vi "RawAttrMap.vi"() -> (3 "AttrMap":T1)   [LabVIEW 2019]
uses:
  Typedef/Def-AttrMap.ctl
  Typedef/Def-NameMap.ctl
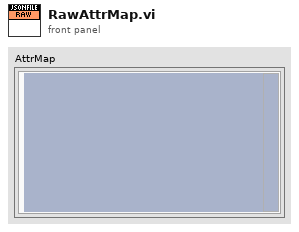
[diagram p1: front panel]
types:
  T1 = typedef "Def-AttrMap.ctl" = cluster{"Map":variant}
  T2 = typedef "Def-NameMap.ctl" = variant[]
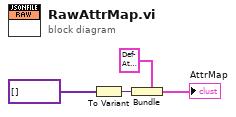
[diagram p0: block diagram]
diagram:
  n1 = To Variant(anything=T2 []) -> (Variant=w4:variant)
  n2 = Bundle(cluster=T1 {"Map"=variant} ("AttrMap"), "Map"=w4) -> (→"AttrMap":T1)
